vi "Is Naughty SubVI.vi"(10 "GObj Refnum":refnum<vi>) -> (1 "SubVI":string, 2 "Naughty SubVI":bool, 3 "VIPath":path, 5 "Is SubVI":bool)   [LabVIEW 2024, in "Wordle Scorer.lvlib"]
uses:
  Wordle Scorer.lvlib
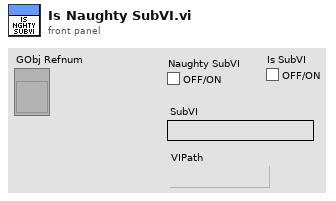
[diagram p1: front panel]
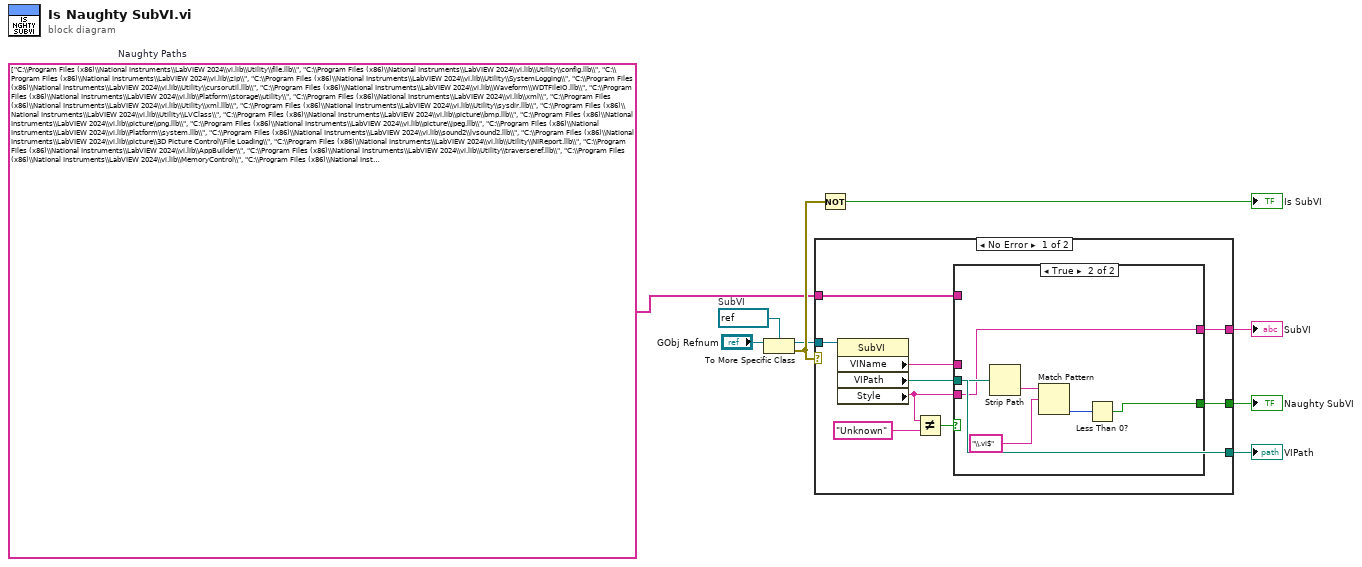
[diagram p0: block diagram]
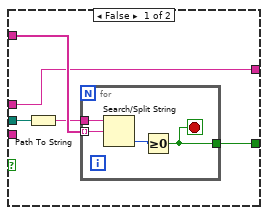
[diagram p2: hidden frame]
diagram:
  w2 = string[] ["C:\\Program Files (x86)\\National Instruments\\LabVIEW 2024\\vi.lib\\Utility\\file.llb\\", "C:\\Program Files (x86)\\National Instruments\\LabVIEW 2024\\vi.lib\\Utility\\config.llb\\", "C:\\Program Files (x86)\\National Instruments\\LabVIEW 2024\\vi.lib\\zip\\", "C:\\Program Files (x86)\\National Instruments\\LabVIEW 2024\\vi.lib\\Utility\\SystemLogging\\", "C:\\Program Files (x86)\\National Instruments\\LabVIEW 2024\\vi.lib\\Utility\\cursorutil.llb\\", "C:\\Program Files (x86)\\National Instruments\\LabVIEW 2024\\vi.lib\\Waveform\\WDTFileIO.llb\\", "C:\\Program Files (x86)\\National Instruments\\LabVIEW 2024\\vi.lib\\Platform\\storage\\utility\\", "C:\\Program Files (x86)\\National Instruments\\LabVIEW 2024\\vi.lib\\xml\\", "C:\\Program Files (x86)\\National Instruments\\LabVIEW 2024\\vi.lib\\Utility\\xml.llb\\", "C:\\Program Files (x86)\\National Instruments\\LabVIEW 2024\\vi.lib\\Utility\\sysdir.llb\\", "C:\\Program Files (x86)\\National Instruments\\LabVIEW 2024\\vi.lib\\Utility\\LVClass\\", "C:\\Program Files (x86)\\National Instruments\\LabVIEW 2024\\vi.lib\\picture\\bmp.llb\\", "C:\\Program Files (x86)\\National Instruments\\LabVIEW 2024\\vi.lib\\picture\\png.llb\\", "C:\\Program Files (x86)\\National Instruments\\LabVIEW 2024\\vi.lib\\picture\\jpeg.llb\\", "C:\\Program Files (x86)\\National Instruments\\LabVIEW 2024\\vi.lib\\Platform\\system.llb\\", "C:\\Program Files (x86)\\National Instruments\\LabVIEW 2024\\vi.lib\\sound2\\lvsound2.llb\\", "C:\\Program Files (x86)\\National Instruments\\LabVIEW 2024\\vi.lib\\picture\\3D Picture Control\\File Loading\\", "C:\\Program Files (x86)\\National Instruments\\LabVIEW 2024\\vi.lib\\Utility\\NIReport.llb\\", "C:\\Program Files (x86)\\National Instruments\\LabVIEW 2024\\vi.lib\\AppBuilder\\", "C:\\Program Files (x86)\\National Instruments\\LabVIEW 2024\\vi.lib\\Utility\\traverseref.llb\\", "C:\\Program Files (x86)\\National Instruments\\LabVIEW 2024\\vi.lib\\MemoryControl\\", "C:\\Program Files (x86)\\National Instruments\\LabVIEW 2024\\vi.lib\\Palette API\\", "C:\\Program Files (x86)\\National Instruments\\LabVIEW 2024\\vi.lib\\Utility\\Get Command Line Arguments.vi", "C:\\Program Files\\NI\\LVAddons\\viawin\\1\\vi.lib\\addons\\analyzer\\analyzerapi.llb\\", "C:\\Program Files\\NI\\LVAddons\\utf32\\1\\vi.lib\\utf\\", "C:\\Program Files (x86)\\National Instruments\\LabVIEW 2024\\vi.lib\\Utility\\LVLibp\\", "C:\\Program Files (x86)\\National Instruments\\LabVIEW 2024\\vi.lib\\Utility\\libraryn.llb\\", "C:\\Program Files (x86)\\National Instruments\\LabVIEW 2024\\vi.lib\\security\\Message Digest\\", "C:\\Program Files (x86)\\National Instruments\\LabVIEW 2024\\vi.lib\\Utility\\file.llb\\", "C:\\Program Files (x86)\\National Instruments\\LabVIEW 2024\\vi.lib\\Platform\\dataskt.llb\\", "C:\\Program Files (x86)\\National Instruments\\LabVIEW 2024\\vi.lib\\Utility\\Resolve Machine Alias.vi", "C:\\Program Files (x86)\\National Instruments\\LabVIEW 2024\\vi.lib\\Utility\\tcp.llb\\", "C:\\Program Files (x86)\\National Instruments\\LabVIEW 2024\\vi.lib\\Instr\\_visa.llb\\", "C:\\Program Files (x86)\\National Instruments\\LabVIEW 2024\\vi.lib\\Platform\\Bluetooth.llb\\", "C:\\Program Files (x86)\\National Instruments\\LabVIEW 2024\\vi.lib\\smtpClient\\", "C:\\Program Files (x86)\\National Instruments\\LabVIEW 2024\\vi.lib\\httpClient\\", "C:\\Program Files (x86)\\National Instruments\\LabVIEW 2024\\vi.lib\\FTP\\", "C:\\Program Files (x86)\\National Instruments\\LabVIEW 2024\\vi.lib\\WebDAVClient\\", "C:\\Program Files (x86)\\National Instruments\\LabVIEW 2024\\vi.lib\\net\\", "C:\\Program Files (x86)\\National Instruments\\LabVIEW 2024\\vi.lib\\SourceControl\\", "C:\\Program Files (x86)\\National Instruments\\LabVIEW 2024\\vi.lib\\wsapi\\", "C:\\Program Files (x86)\\National Instruments\\LabVIEW 2024\\vi.lib\\Platform\\dotnet.llb\\", "C:\\Program Files (x86)\\National Instruments\\LabVIEW 2024\\vi.lib\\Utility\\inputDevices.llb\\", "C:\\Program Files (x86)\\National Instruments\\LabVIEW 2024\\vi.lib\\registry\\", "C:\\Program Files (x86)\\National Instruments\\LabVIEW 2024\\vi.lib\\Python\\", "C:\\Program Files\\NI\\LVAddons\\dct\\1\\vi.lib\\addons\\database\\", "C:\\Program Files\\NI\\LVAddons\\dfc\\1\\vi.lib\\DataFinder\\", "C:\\Program Files (x86)\\National Instruments\\LabVIEW 2024\\vi.lib\\MakerHub\\", "C:\\Program Files\\NI\\LVAddons\\nisyscfg\\1\\vi.lib\\nisyscfg\\"]  # Naughty Paths
  w7 = refnum<vi> refnum  # SubVI
  n1 = To More Specific Class(target class=w7, reference="GObj Refnum") -> (specific class reference=w6:refnum<vi>, error out=w9:errorcluster)  [unwired: 1 in]
  n2 = case shown="No Error" w9 {
    tunnel: w6 -> [w18 _]
    tunnel: [w17 _] -> w5
    tunnel: [w10 _] -> w4
    tunnel: [w16 _] -> w3
    tunnel: w2 -> [w15 _]
    frame No Error {
      n3 = property class="SubVI"(reference=w18) -> ("VIName"=w12:string, "VIPath"=w16:path, "Style"=w11:string)  [unwired: 1 in, 2 out]
      n4 = Not Equal?(x=w11, y="Unknown") -> (x != y?=w13:bool)
      n5 = case shown="True" w13 {
        tunnel: [w23 w29] -> w17
        tunnel: w16 -> [w22 w31]
        tunnel: w15 -> [w21 _]
        tunnel: w12 -> [w19 _]
        tunnel: w11 -> [_ w28]
        tunnel: [w19 w28] -> w10
        frame False {
          n6 = Path To String(path=w22) -> (string=w20:string)
          n7 = for {
            tunnel: w20 -> [w26]
            tunnel: [w27] -> w23
            tunnel: w21 -> [w25] mode=indexing
            stop <- w27 stop-if-true
            n8 = Search/Split String(string=w26, search string/char (-)=w25) -> (offset of match=w24:i32)  [unwired: 1 in, 2 out]
            n9 = Greater Or Equal To 0?(x=w24) -> (x >= 0?=w27:bool)
          }
        }
        frame True {
          n10 = Strip Path(path=w31) -> (name=w30:string)  [unwired: 1 out]
          n11 = Match Pattern(string=w30, regular expression="\\.vi$") -> (offset past match=w32:i32)  [unwired: 1 in, 3 out]
          n12 = Less Than 0?(x=w32) -> (x < 0?=w29:bool)
        }
      }
    }
    frame Error {
    }
  }
  "Naughty SubVI" <- w5
  "SubVI" <- w4
  "VIPath" <- w3
  n13 = Not(x=w9) -> (.not. x?=→"Is SubVI":bool)
